vi "DHE_DRV_set_destination.vi"(0 "fd":i32, 5 "num of args":i32, 7 "board dest":i32, 11 "error in (no error)":errorcluster) -> (4 "fd out":i32, 8 "return value":i32, 15 "error out":errorcluster)   [LabVIEW 2016]
doc: "This VI closes the I/O interface with the instrument."
uses:
  c/lib/libarcDHE.so
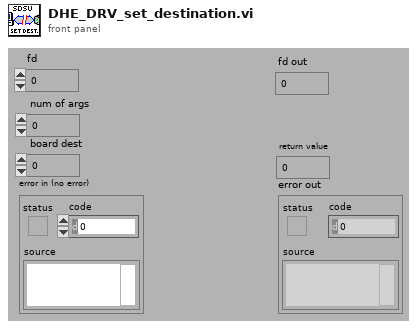
[diagram p1: front panel]
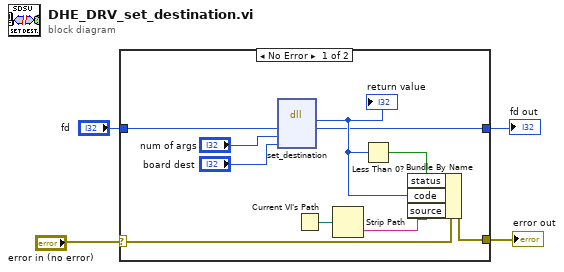
[diagram p0: block diagram]
diagram:
  n1 = case shown="No Error" "error in (no error)" {
    selector: "error in (no error)" -> [w5 w15]
    tunnel: [w10 w15] -> w4
    tunnel: [w7 w16] -> w3
    tunnel: "fd" -> [w6 w16]
    frame No Error {
      n2 = dll-call lib="home/simager/panview/PAN/Modules/SDSU/private/c/lib/libarcDHE.so" fn="set_destination"("fd"=w6, "num_of_args"="num of args", "board_dest"="board dest") -> (w13:i32, "fd"=w7:i32)  [unwired: 5 in, 2 out]
      "return value" <- w13
      n3 = Current VI's Path() -> (path=w12:path)
      n4 = Strip Path(path=w12) -> (name=w11:string)  [unwired: 1 out]
      n5 = Less Than 0?(x=w13) -> (x < 0?=w14:bool)
      n6 = Bundle By Name(cluster=w5, "status"=w14, "code"=w13, "source"=w11) -> (w10:errorcluster)
    }
    frame Error {
    }
  }
  "error out" <- w4
  "fd out" <- w3
